vi "data_convert_for_xy_graph.vi"(7 "pulse reset":bool, 8 "data num in":u16, 9 "disp num":u16, 10 "graph data in":T1(array[cluster]), 11 "new data in":T1(array[cluster])) -> (0 "data num out":u16, 1 "min":i64, 2 "max":i64, 3 "data out":T2(array[cluster]))   [LabVIEW 2020]
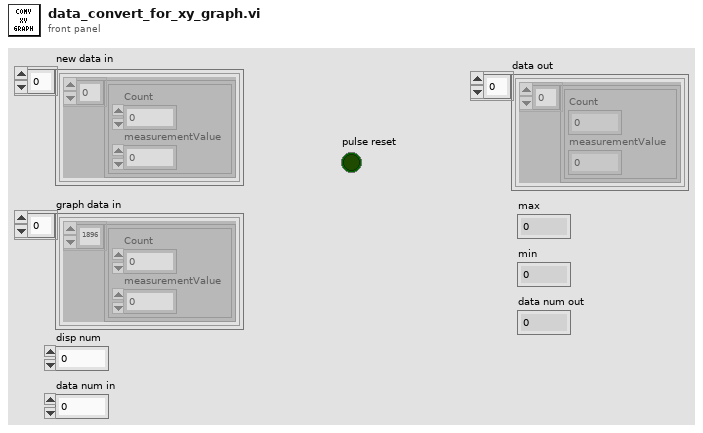
[diagram p1: front panel]
types:
  T1 = cluster{"data":cluster{"Count":dbl, "measurementValue":dbl}[]}[]
  T2 = cluster{cluster{"Count":dbl, "measurementValue":dbl}[]}[]
  T3 = cluster{"data":cluster{"Count":dbl, "measurementValue":dbl}[]}
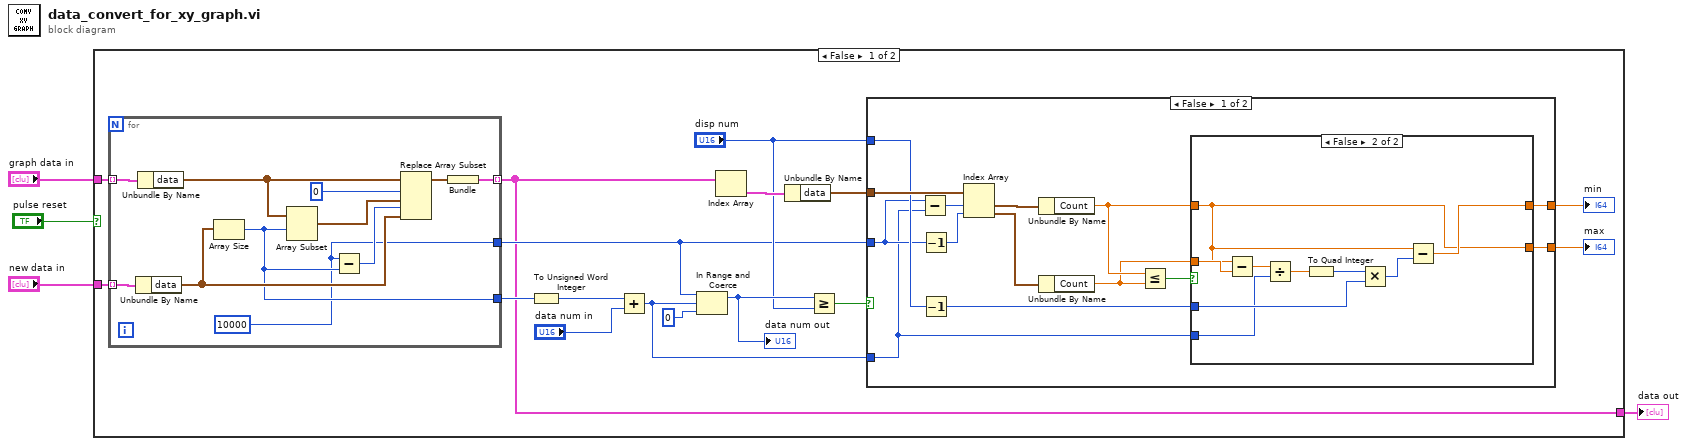
[diagram p0: block diagram]
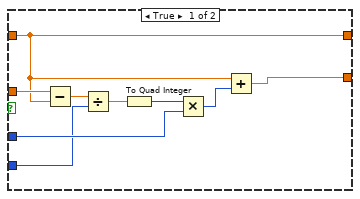
[diagram p2: hidden frame]
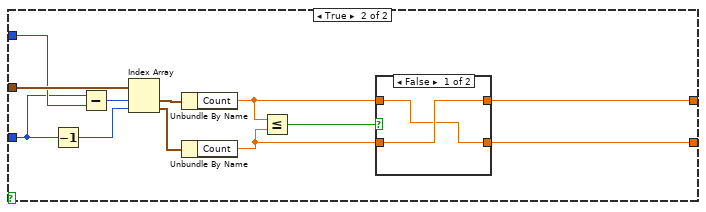
[diagram p3: hidden frame]
diagram:
  n1 = case shown="False" "pulse reset" {
    tunnel: "graph data in" -> [w11 w80]
    tunnel: "new data in" -> [w10 _]
    tunnel: [w5 w80] -> w1
    frame False {
      n2 = for {
        tunnel: w11 -> [w79] mode=indexing
        tunnel: w10 -> [w78] mode=indexing
        tunnel: [w72] -> w5 mode=indexing
        tunnel: [w70] -> w19
        tunnel: [w69] -> w6
        w69 = u16 10000 ("disp num")
        n3 = Unbundle By Name(w78) -> ("data"=w74:cluster{"Count":dbl, "measurementValue":dbl}[])
        n4 = Unbundle By Name(w79) -> ("data"=w77:cluster{"Count":dbl, "measurementValue":dbl}[])
        n5 = Array Size(array=w74) -> (size(s)=w70:i32)
        n6 = Array Subset(array=w77, index=w70) -> (w75:cluster{"Count":dbl, "measurementValue":dbl}[])  [unwired: 1 in]
        n7 = Subtract(x=w69, y=w70) -> (x-y=w71:i32)
        n8 = Replace Array Subset(array=w77, new element #1=w75, index #1=0, new element #2=w74, index #2=w71) -> (w73:cluster{"Count":dbl, "measurementValue":dbl}[])
        n9 = Bundle("data"=w73) -> (w72:T3)  [unwired: 1 in]
      }
      n10 = To Unsigned Word Integer(number=w19) -> (unsigned 16bit integer=w17:u16)
      n11 = Add(x=w17, y="data num in") -> (x+y=w12:u16)
      n12 = In Range and Coerce(upper limit=w6, x=w12, lower limit=u16 0) -> (coerced(x)=w15:u16)  [unwired: 1 out]
      "data num out" <- w15
      n13 = Index Array(array=w5) -> (element=w13:T3)  [unwired: 1 in]
      n14 = Unbundle By Name(w13) -> ("data"=w7:cluster{"Count":dbl, "measurementValue":dbl}[])
      n15 = Greater Or Equal?(x=w15, y="disp num") -> (x >= y?=w14:bool)
      n16 = case shown="False" w14 {
        tunnel: [w31 w53] -> w20
        tunnel: [w29 w54] -> w9
        tunnel: w6 -> [w25 w58]
        tunnel: w7 -> [w34 w61]
        tunnel: w12 -> [w21 _]
        tunnel: "disp num" -> [w30 w60]
        frame False {
          n17 = Subtract(x=w25, y=w21) -> (x-y=w33:u16)
          n18 = Decrement(x=w25) -> (x-1=w24:u16)
          n19 = Decrement(x=w30) -> (x-1=w26:u16)
          n20 = Index Array(array=w34, index #1=w33, index #2=w24) -> (element #1=w32:cluster{"Count":dbl, "measurementValue":dbl}, element #2=w23:cluster{"Count":dbl, "measurementValue":dbl})
          n21 = Unbundle By Name(w32) -> ("Count"=w28:dbl)
          n22 = Unbundle By Name(w23) -> ("Count"=w22:dbl)
          n23 = Less Or Equal?(x=w28, y=w22) -> (x <= y?=w27:bool)
          n24 = case shown="False" w27 {
            tunnel: [w43 w44] -> w31
            tunnel: [w35 w46] -> w29
            tunnel: w28 -> [w35 w44]
            tunnel: w26 -> [w41 w51]
            tunnel: w21 -> [w39 w49]
            tunnel: w22 -> [w36 w45]
            frame True {
              n25 = Subtract(x=w36, y=w35) -> (x-y=w40:dbl)
              n26 = Divide(x=w40, y=w39) -> (x/y=w38:dbl)
              n27 = To Quad Integer(1:w38) -> (0:w37:i64)
              n28 = Multiply(x=w37, y=w41) -> (x*y=w42:i64)
              n29 = Add(x=w35, y=w42) -> (x+y=w43:dbl)
            }
            frame False {
              n30 = Subtract(x=w44, y=w45) -> (x-y=w50:dbl)
              n31 = Divide(x=w50, y=w49) -> (x/y=w48:dbl)
              n32 = To Quad Integer(1:w48) -> (0:w47:i64)
              n33 = Multiply(x=w47, y=w51) -> (x*y=w52:i64)
              n34 = Subtract(x=w44, y=w52) -> (x-y=w46:dbl)
            }
          }
        }
        frame True {
          n35 = Decrement(x=w58) -> (x-1=w62:u16)
          n36 = Subtract(x=w58, y=w60) -> (x-y=w59:u16)
          n37 = Index Array(array=w61, index #1=w59, index #2=w62) -> (element #1=w64:cluster{"Count":dbl, "measurementValue":dbl}, element #2=w63:cluster{"Count":dbl, "measurementValue":dbl})
          n38 = Unbundle By Name(w64) -> ("Count"=w55:dbl)
          n39 = Unbundle By Name(w63) -> ("Count"=w56:dbl)
          n40 = Less Or Equal?(x=w55, y=w56) -> (x <= y?=w57:bool)
          n41 = case shown="False" w57 {
            tunnel: w56 -> [w66 w67]
            tunnel: w55 -> [w65 w68]
            tunnel: [w66 w68] -> w54
            tunnel: [w65 w67] -> w53
            frame False {
            }
            frame True {
            }
          }
        }
      }
      "min" <- w9
      "max" <- w20
    }
    frame True {
    }
  }
  "data out" <- w1
